vi "Brute Force Measurment SubVI Posibly Modded For Trip Prevention System.vi"(8 "error in (no error)":errorcluster, 9 "BoardHandle in":T1, 10 "Stop Program Brute Force":bool, 11 "Barcodes in":string[](array[string])) -> (0 "error out":errorcluster, 1 "BoardHandle out":T1, 2 "Actual Voltage Level (V) 2":dbl format="%#_13g", 4 "channel 4 currents":dbl[](array[numeric]), 5 "channel 2 currents":dbl[](array[numeric]), 6 "channel 3 currents":dbl[](array[numeric]), 7 "channel 1 currents":dbl[](array[numeric]))   [LabVIEW 2020]
panel:
  # "INPUT"
  # "OUTPUT"
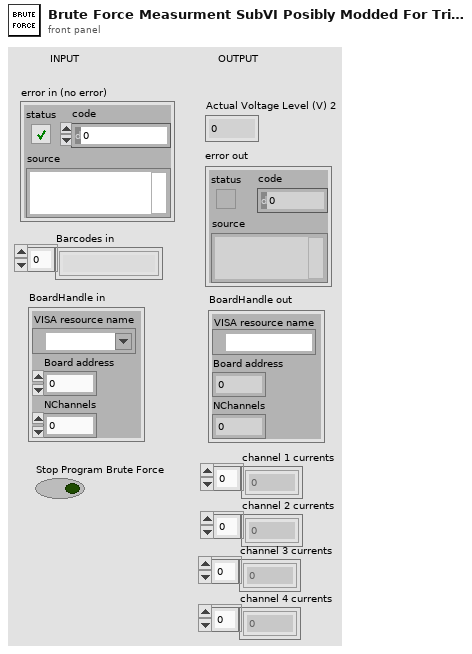
[diagram p1: front panel]
types:
  T1 = cluster{"VISA resource name":refnum<visa-resource-name>, "Board address":u8, "NChannels":u8}
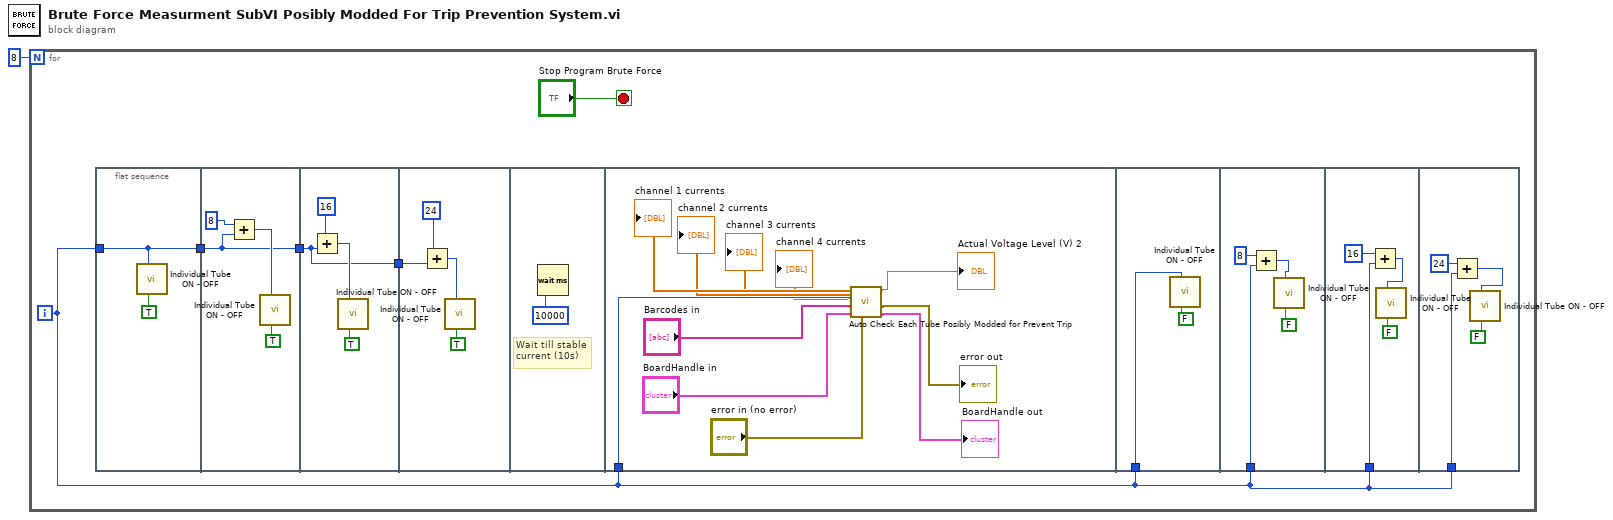
[diagram p0: block diagram]
diagram:
  n1 = for {
    N: 8 -> [_]
    i -> [w2]
    stop <- "Stop Program Brute Force" stop-if-true
    n2 = flat-sequence {
      tunnel: w2 -> [w7]
      tunnel: [w7] -> w5
      tunnel: w5 -> [w10]
      tunnel: [w10] -> w4
      tunnel: w4 -> [w14]
      tunnel: [w14] -> w3
      tunnel: w3 -> [w18]
      tunnel: w2 -> [w29]
      tunnel: w2 -> [w34]
      tunnel: w2 -> [w37]
      tunnel: w2 -> [w41]
      tunnel: w2 -> [w45]
      frame #0 {
        n3 = call "Individual Tube ON - OFF.vi"("Single Tube ON/OFF"=TRUE, "Tube #"=w7) -> ()  [unwired: 10 in]
      }
      frame #1 {
        n4 = Add(x=8, y=w10) -> (x+y=w12:i32)
        n5 = call "Individual Tube ON - OFF.vi"("Single Tube ON/OFF"=TRUE, "Tube #"=w12) -> ()  [unwired: 10 in]
      }
      frame #2 {
        n6 = Add(x=16, y=w14) -> (x+y=w16:i32)
        n7 = call "Individual Tube ON - OFF.vi"("Single Tube ON/OFF"=TRUE, "Tube #"=w16) -> ()  [unwired: 10 in]
      }
      frame #3 {
        n8 = Add(x=24, y=w18) -> (x+y=w20:i32)
        n9 = call "Individual Tube ON - OFF.vi"("Single Tube ON/OFF"=TRUE, "Tube #"=w20) -> ()  [unwired: 10 in]
      }
      frame #4 {
        # "Wait till stable\ncurrent (10s)"
        n10 = Wait (ms)(milliseconds to wait=u32 10000) -> ()  [unwired: 1 out]
      }
      frame #5 {
        n11 = call "Auto Check Each Tube Posibly Modded for Prevent Trip.vi"("error in (no error)"="error in (no error)", "BoardHandle in"="BoardHandle in", "Barcodes in"="Barcodes in", "Tube #"=w29) -> ("BoardHandle out"=→"BoardHandle out":T1, "error out"=→"error out":errorcluster, "channel 4 currents"=→"channel 4 currents":dbl[], "Actual Voltage Level (V) 2"=→"Actual Voltage Level (V) 2":dbl, "channel 3 currents"=→"channel 3 currents":dbl[], "channel 2 currents"=→"channel 2 currents":dbl[], "channel 1 currents"=→"channel 1 currents":dbl[])  [unwired: 1 in]
      }
      frame #6 {
        n12 = call "Individual Tube ON - OFF.vi"("Single Tube ON/OFF"=FALSE, "Tube #"=w34) -> ()  [unwired: 10 in]
      }
      frame #7 {
        n13 = Add(x=8, y=w37) -> (x+y=w38:i32)
        n14 = call "Individual Tube ON - OFF.vi"("Single Tube ON/OFF"=FALSE, "Tube #"=w38) -> ()  [unwired: 10 in]
      }
      frame #8 {
        n15 = Add(x=16, y=w41) -> (x+y=w42:i32)
        n16 = call "Individual Tube ON - OFF.vi"("Single Tube ON/OFF"=FALSE, "Tube #"=w42) -> ()  [unwired: 10 in]
      }
      frame #9 {
        n17 = Add(x=24, y=w45) -> (x+y=w46:i32)
        n18 = call "Individual Tube ON - OFF.vi"("Single Tube ON/OFF"=FALSE, "Tube #"=w46) -> ()  [unwired: 10 in]
      }
    }
  }
